vi "Wait-for-action.vi"(8 "error in (no error)":errorcluster, 11 "Object ref in":T2) -> (0 "error out":errorcluster, 2 "Next action":T1, 3 "Object ref out":T2)   [LabVIEW 2013, in "SLMControl.lvlib" / "SC-Main.lvclass"]
uses:
  SC-Main.lvclass
  Object-reference.ctl
  Main-actions.ctl
  SC-Main.lvclass/SC-Main.ctl
  Read Action queue.vi
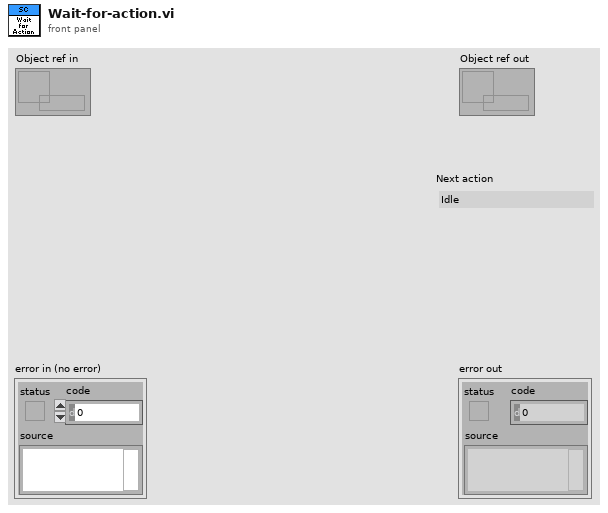
[diagram p1: front panel]
types:
  T1 = typedef "SLMControl.lvlib/SC-Main.lvclass/Main-actions.ctl" = enum16{"Idle", "Initialize", "Load configuration", "Save configuration", "Load lasing files", "Load deposition files", "Refresh files", "Clear files", "Open lasing file", "Activate", "Start", "Start deposition cycle", "Start lasing cycle", "Iterate", "Abort", "Stop", "Exit"}
  T2 = typedef "SLMControl.lvlib/SC-Main.lvclass/Object-reference.ctl" = refnum<data-value>
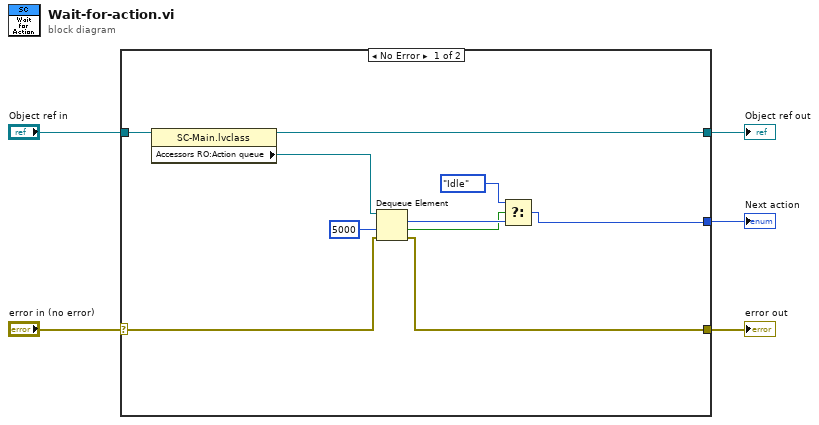
[diagram p0: block diagram]
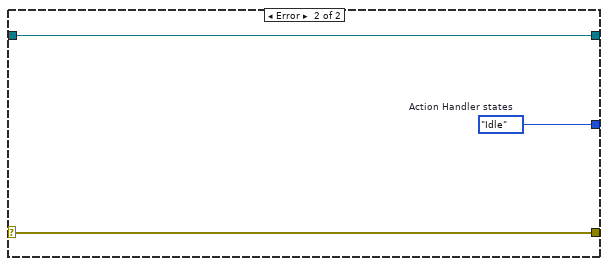
[diagram p2: hidden frame]
diagram:
  n1 = case shown="No Error" "error in (no error)" {
    selector: "error in (no error)" -> [w13 w18]
    tunnel: [w12 w18] -> w4
    tunnel: [w14 w17] -> w2
    tunnel: "Object ref in" -> [w15 w17]
    tunnel: [w7 w16] -> w1
    frame No Error {
      n2 = property class="SC-Main.lvclass"(reference=w15) -> (reference out=w14:T2, "Accessors RO:Action queue"=w6:refnum<queue>)  [unwired: 1 in, 1 out]
      n3 = Dequeue Element(queue=w6, timeout in ms (-1)=5000, error in (no error)=w13) -> (element=w10:T1, timed out?=w9:bool, error out=w12:errorcluster)  [unwired: 1 out]
      n4 = Select(t=Main-actions."Idle" ("Next action"), s=w9, f=w10) -> (s? t:f=w7:T1)
    }
    frame Error {
      w16 = Main-actions."Idle"  # Action Handler states
    }
  }
  "error out" <- w4
  "Object ref out" <- w2
  "Next action" <- w1
